vi "Property_Tree Tag_Parse Property Name.vi"(11 "Tag Property Name":string="Terminal.Wire.Position:Left") -> (0 "Parent":string, 1 "Display name short":string, 2 "Display name":string, 3 "Parent Array":string[](array[string]))   [LabVIEW 2023]
panel:
  out "Property Hierarchy":string[](array[string])
  # "Parent is relevant to the tree, not necessarily to the property hierarchy"
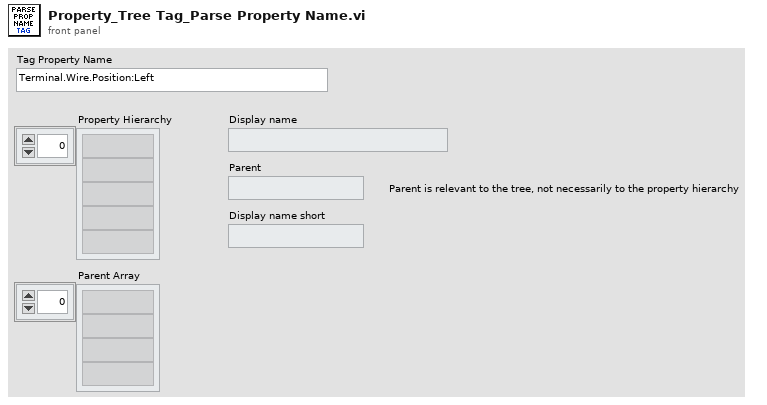
[diagram p1: front panel]
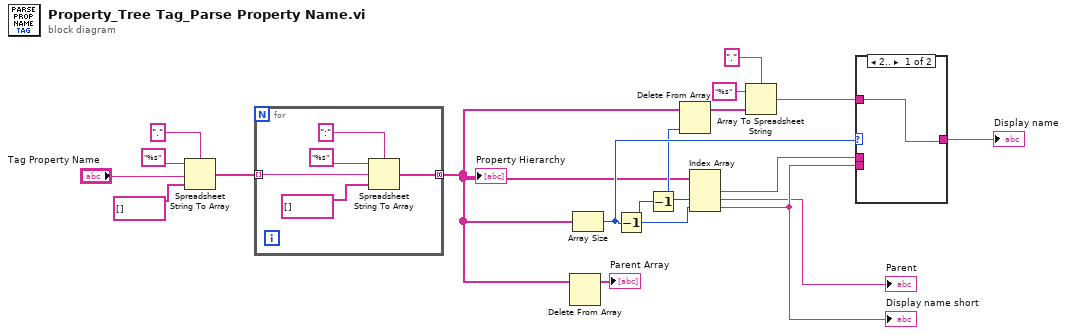
[diagram p0: block diagram]
diagram:
  n1 = Spreadsheet String To Array(delimiter (Tab)=".", format string="%s" ("delimiter (Tab)"), spreadsheet string="Tag Property Name", array type (2D Dbl)=string[] [] ("delimiter (Tab)")) -> (array=w14:string[])
  n2 = for {
    tunnel: w14 -> [w20] mode=indexing
    tunnel: [w19] -> w2 mode=concatenating
    n3 = Spreadsheet String To Array(delimiter (Tab)=":", format string="%s" ("delimiter (Tab)"), spreadsheet string=w20, array type (2D Dbl)=string[] [] ("delimiter (Tab)")) -> (array=w19:string[])
  }
  "Property Hierarchy" <- w2
  n4 = Delete From Array(array=w2) -> (array with subset deleted=→"Parent Array":string[])  [unwired: 2 in, 1 out]
  n5 = Array Size(array=w2) -> (size(s)=w9:i32)
  n6 = Decrement(x=w9) -> (x-1=w5:i32)
  n7 = Decrement(x=w5) -> (x-1=w3:i32)
  n8 = Delete From Array(array=w2, index=w3) -> (array with subset deleted=w8:string[])  [unwired: 1 in, 1 out]
  n9 = Index Array(array=w2, index #2=w3, index #3=w5) -> (element #1=w10:string, element #2=→"Parent":string, element #3=w12:string)  [unwired: 1 in]
  "Display name short" <- w12
  n10 = Array To Spreadsheet String(delimiter (Tab)=".", array=w8, 3:"%s" ("format string")) -> (spreadsheet string=w4:string)
  n11 = case shown="2.." w9 {
    tunnel: w10 -> [_ _]
    tunnel: [w24 w25] -> w13
    tunnel: w12 -> [_ w25]
    tunnel: w4 -> [w24 _]
    frame 2.. {
    }
    frame 1, Default {
    }
  }
  "Display name" <- w13
